vi "Test Number To Column Letter.vi"(11 "Test Case In":refnum<class "Test Open Xml.lvclass">) -> (0 "error out":errorcluster, 3 "Test Case Out":refnum<class "Test Open Xml.lvclass">)   [LabVIEW 2021, in "Test Open Xml.lvclass"]
uses:
  Test Open Xml.lvclass
  C:/Program Files/National Instruments/LabVIEW 2025/vi.lib/Astemes/LUnit/Test Case.lvclass
  <vilib>/Astemes/LUnit/Test Case.lvclass/Test Case.ctl
  Test Open Xml.lvclass/Test Open Xml.ctl
  <vilib>/Astemes/LUnit/Test Case.lvclass
  Source/Open Xml.lvlib
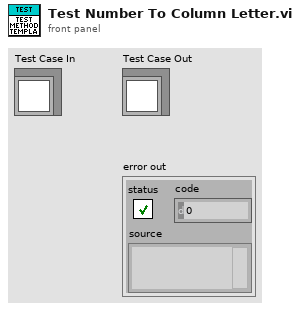
[diagram p1: front panel]
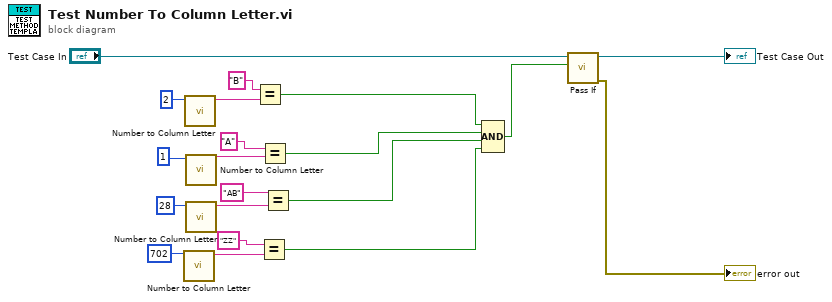
[diagram p0: block diagram]
diagram:
  n1 = call "Number to Column Letter.vi"("Number"=702 ("x")) -> ("String"=w3:string)  [unwired: 10 in]
  n2 = call "Number to Column Letter.vi"("Number"=2 ("x")) -> ("String"=w6:string)  [unwired: 10 in]
  n3 = call "Number to Column Letter.vi"("Number"=1 ("x")) -> ("String"=w5:string)  [unwired: 10 in]
  n4 = call "Number to Column Letter.vi"("Number"=28 ("x")) -> ("String"=w1:string)  [unwired: 10 in]
  n5 = Equal?(x="B", y=w6) -> (x = y?=w17:bool)
  n6 = Equal?(x="ZZ" ("Letter"), y=w3) -> (x = y?=w14:bool)
  n7 = Equal?(x="A", y=w5) -> (x = y?=w16:bool)
  n8 = Equal?(x="AB", y=w1) -> (x = y?=w15:bool)
  n9 = Compound Arithmetic op=AND(w17, w16, w15, w14) -> (w13:bool)
  n10 = call <vilib>:"Pass If.vi"("Pass?"=w13, "LUnit Test Case In"="Test Case In") -> ("error out"=→"error out":errorcluster, "LUnit Test Case Out"=→"Test Case Out":refnum<class "Test Open Xml.lvclass">)  [unwired: 8 in]
